vi "Switch_DataLog.vi"() -> ()   [LabVIEW 2016]
uses:
  MGCC_DataLog_global.vi
  Finite State Machine (He Yin)/Sub-VIs/MGCC_FntStaMach_gobal.vi
  Global tdms reference.vi
  Communication/Global communication.vi
  Model Management (He Yin)/Global_MdlMgmt.vi
  <vilib>/Utility/error.llb/Error Cluster From Error Code.vi
  <vilib>/ErrorRing/Error Ring.xnode
panel:
  in  "Start 3":bool=TRUE
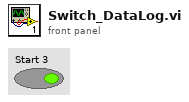
[diagram p1: front panel]
types:
  T1 = enum16{"open", "open or create", "create or replace", "create", "open (read-only)"}
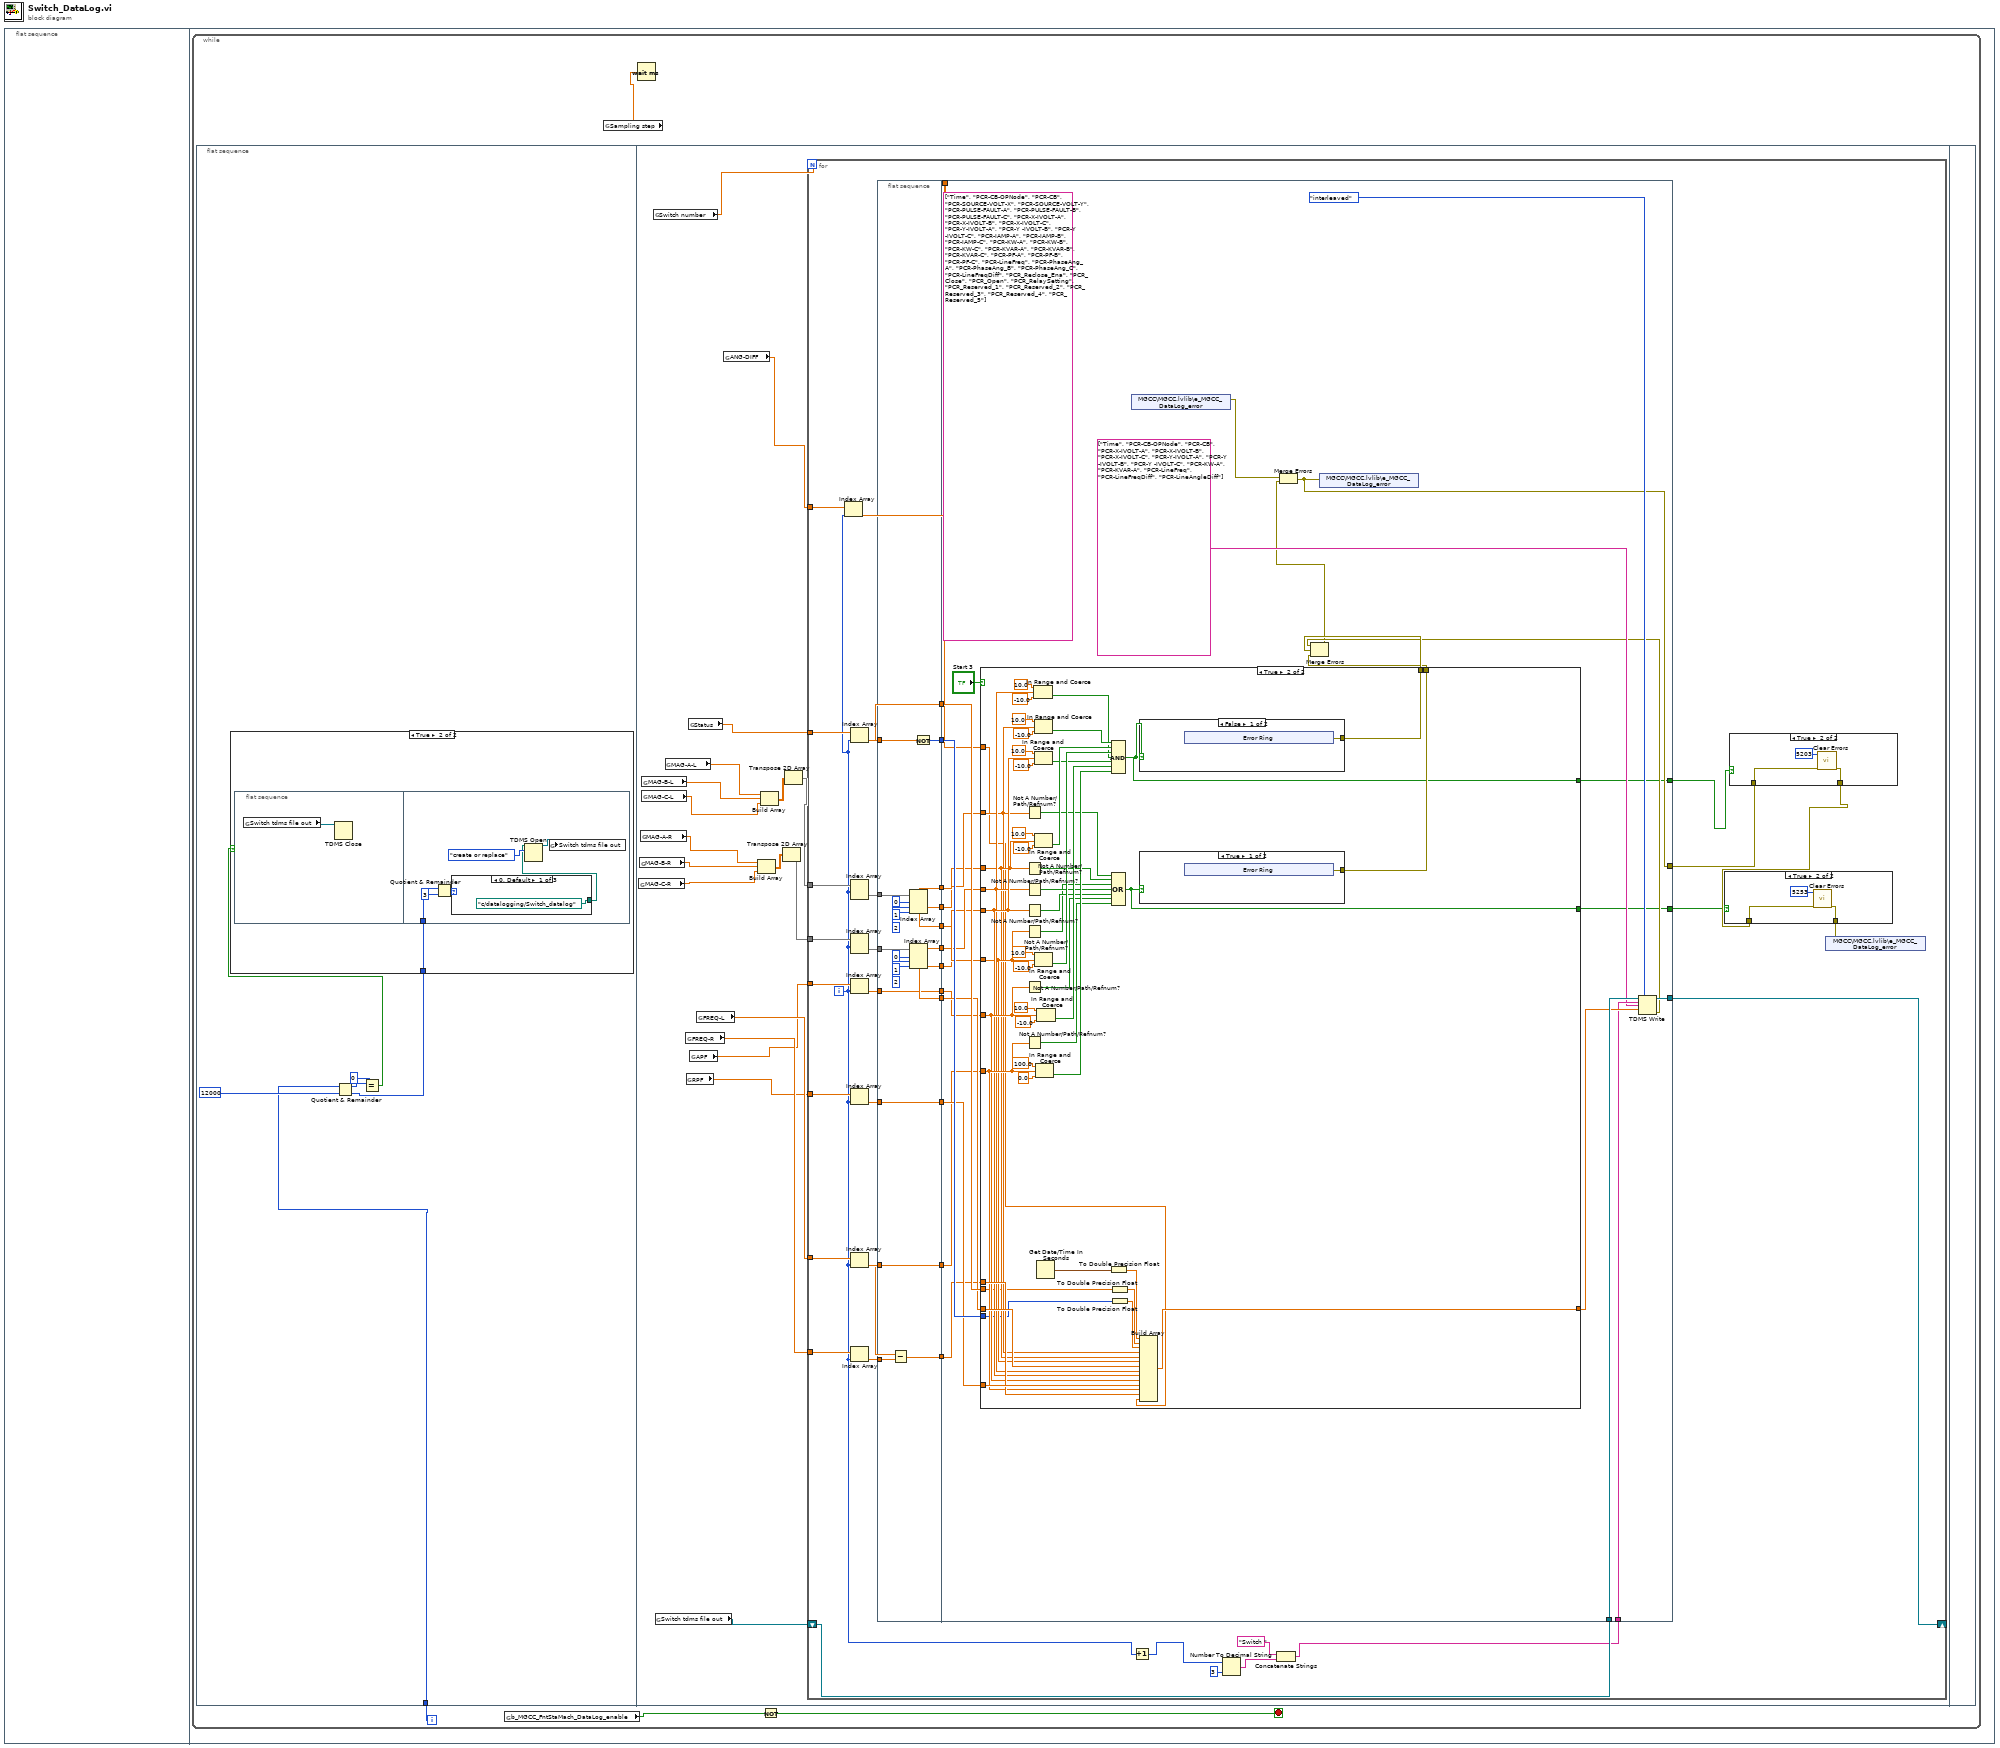
[diagram p0: block diagram]
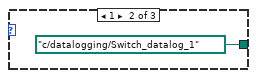
[diagram p3: hidden frame]
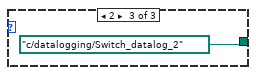
[diagram p4: hidden frame]
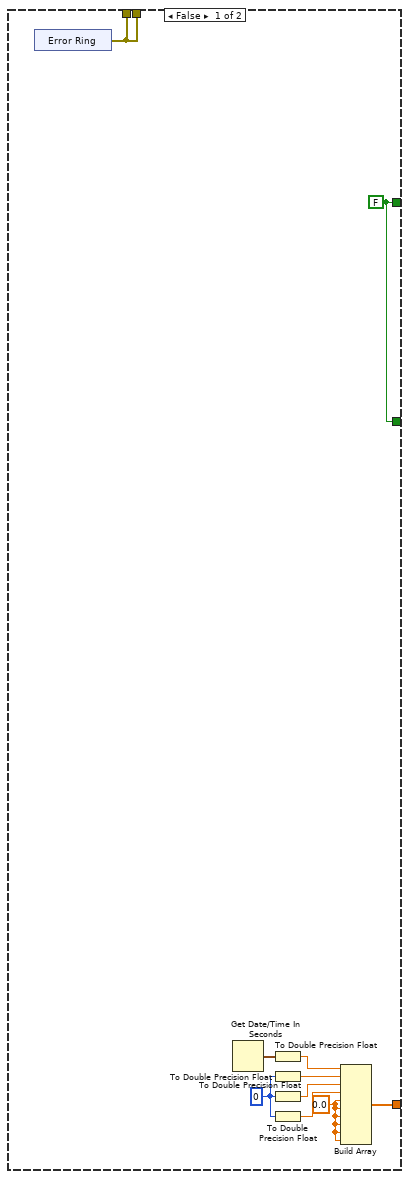
[diagram p7: hidden frame]
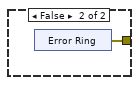
[diagram p8: hidden frame]
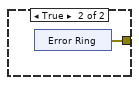
[diagram p9: hidden frame]
diagram:
  n1 = flat-sequence {
    frame #0 {
    }
    frame #1 {
      n2 = while {
        i -> [w2]
        stop <- w4 stop-if-true
        n3 = flat-sequence {
          tunnel: w2 -> [w5]
          frame #0 {
            n4 = Quotient & Remainder(x=w5, y=12000) -> (x-y*floor(x/y)=w9:i32, floor(x/y)=w6:i32)
            n5 = Equal?(x=w9, y=0) -> (x = y?=w7:bool)
            n6 = case shown="True" w7 {
              tunnel: w6 -> [_ w11]
              frame False {
              }
              frame True {
                n7 = flat-sequence {
                  tunnel: w11 -> [w16]
                  frame #0 {
                    n8 = global read "Global tdms reference.vi" "Switch tdms file out"() -> (w12:refnum<k34>)
                    n9 = TDMS Close(11:w12) -> ()  [unwired: 1 in, 2 out]
                  }
                  frame #1 {
                    n10 = Quotient & Remainder(x=w16, y=3) -> (x-y*floor(x/y)=w14:i32)  [unwired: 1 out]
                    n11 = case shown="0, Default" w14 {
                      tunnel: [path "c:/datalogging/Switch_datalog" ("file path (dialog if empty)") path "c:/datalogging/Switch_datalog_1" ("file path (dialog if empty)") path "c:/datalogging/Switch_datalog_2" ("file path (dialog if empty)")] -> w13
                      frame 0, Default {
                      }
                      frame 1 {
                      }
                      frame 2 {
                      }
                    }
                    n12 = TDMS Open(10:T1."create or replace" ("operation (0:open)"), 11:w13) -> (3:w18:refnum<k34>)  [unwired: 5 in, 1 out]
                    n13 = global write "Global tdms reference.vi" "Switch tdms file out"(w18) -> ()
                  }
                }
              }
            }
          }
          frame #1 {
            n14 = global read "Global communication.vi" "MAG-C-R"() -> (w26:dbl[])
            n15 = global read "Global communication.vi" "MAG-B-R"() -> (w27:dbl[])
            n16 = global read "Global communication.vi" "MAG-A-R"() -> (w28:dbl[])
            n17 = global read "Global communication.vi" "MAG-B-L"() -> (w24:dbl[])
            n18 = global read "Global communication.vi" "MAG-C-L"() -> (w23:dbl[])
            n19 = global read "Global_MdlMgmt.vi" "Switch number"() -> (w22:dbl)
            n20 = global read "Global tdms reference.vi" "Switch tdms file out"() -> (w39:refnum<k34>)
            n21 = global read "Global communication.vi" "MAG-A-L"() -> (w25:dbl[])
            n22 = global read "Global communication.vi" "FREQ-R"() -> (w31:dbl[])
            n23 = global read "Global communication.vi" "RPF"() -> (w29:dbl[])
            n24 = global read "Global communication.vi" "Status"() -> (w33:dbl[])
            n25 = global read "Global communication.vi" "APF"() -> (w30:dbl[])
            n26 = global read "Global communication.vi" "FREQ-L"() -> (w32:dbl[])
            n27 = global read "Global communication.vi" "ANG-DIFF"() -> (w34:dbl[])
            n28 = Build Array(w28, w27, w26) -> (w36:dbl[][])
            n29 = Build Array(w25, w24, w23) -> (w38:dbl[][])
            n30 = Transpose 2D Array(2D array=w36) -> (transposed array=w35:dbl[][])
            n31 = Transpose 2D Array(2D array=w38) -> (transposed array=w37:dbl[][])
            n32 = for {
              N: w22 -> [_]
              tunnel: w33 -> [w78]
              tunnel: w37 -> [w74]
              tunnel: w35 -> [w72]
              tunnel: w30 -> [w68]
              tunnel: w29 -> [w70]
              tunnel: w32 -> [w66]
              tunnel: w31 -> [w76]
              shift-right: [w79] -> _
              shift-left: w39 -> [w80]
              tunnel: w34 -> [w50]
              i -> [w44]
              n33 = Index Array(array=w50, index=w44) -> (element=w49:dbl)
              n34 = Index Array(array=w78, index=w44) -> (element=w77:dbl)
              n35 = Index Array(array=w74, index (row)=w44) -> (element=w73:dbl[])  [unwired: 1 in]
              n36 = Index Array(array=w72, index (row)=w44) -> (element=w71:dbl[])  [unwired: 1 in]
              n37 = Index Array(array=w68, index=w44) -> (element=w67:dbl)
              n38 = Index Array(array=w70, index=w44) -> (element=w69:dbl)
              n39 = Index Array(array=w66, index=w44) -> (element=w65:dbl)
              n40 = Index Array(array=w76, index=w44) -> (element=w75:dbl)
              n41 = flat-sequence {
                tunnel: w77 -> [w100]
                tunnel: w73 -> [w109]
                tunnel: w71 -> [w102]
                tunnel: w67 -> [w92]
                tunnel: w69 -> [w91]
                tunnel: w65 -> [w90]
                tunnel: w75 -> [w101]
                tunnel: [w100] -> w64
                tunnel: [w99] -> w63
                tunnel: [w98] -> w62
                tunnel: [w97] -> w61
                tunnel: [w96] -> w60
                tunnel: [w95] -> w59
                tunnel: [w94] -> w58
                tunnel: [w93] -> w57
                tunnel: [w92] -> w56
                tunnel: [w91] -> w55
                tunnel: [w90] -> w54
                tunnel: [w89] -> w53
                tunnel: w80 -> [w136]
                tunnel: w45 -> [w133]
                tunnel: [w132] -> w79
                tunnel: w64 -> [w131]
                tunnel: w63 -> [w130]
                tunnel: w62 -> [w129]
                tunnel: w61 -> [w128]
                tunnel: w60 -> [w127]
                tunnel: w59 -> [w126]
                tunnel: w58 -> [w125]
                tunnel: w57 -> [w124]
                tunnel: w56 -> [w123]
                tunnel: w55 -> [w122]
                tunnel: w54 -> [w121]
                tunnel: w53 -> [w120]
                tunnel: [w113] -> w52
                tunnel: [w112] -> w51
                tunnel: w49 -> [w111]
                tunnel: [w110] -> w40
                frame #0 {
                  n42 = Subtract(x=w90, y=w101) -> (x-y=w89:dbl)
                  n43 = Index Array(array=w109, index #1=0 ("index"), index #2=1 ("index"), index #3=2 ("index")) -> (element #1=w98:dbl, element #2=w97:dbl, element #3=w96:dbl)
                  n44 = Index Array(array=w102, index #1=0 ("index"), index #2=1 ("index"), index #3=2 ("index")) -> (element #1=w95:dbl, element #2=w94:dbl, element #3=w93:dbl)
                  n45 = Not(x=w100) -> (.not. x?=w99:u32)
                }
                frame #1 {
                  (unwired) string[] ["Time", "PCR-CB-OPNode", "PCR-CB", "PCR-SOURCE-VOLT-X", "PCR-SOURCE-VOLT-Y", "PCR-PULSE-FAULT-A", "PCR-PULSE-FAULT-B", "PCR-PULSE-FAULT-C", "PCR-X-IVOLT-A", "PCR-X-IVOLT-B", "PCR-X-IVOLT-C", "PCR-Y-IVOLT-A", "PCR-Y -IVOLT-B", "PCR-Y -IVOLT-C", "PCR-IAMP-A", "PCR-IAMP-B", "PCR-IAMP-C", "PCR-KW-A", "PCR-KW-B", "PCR-KW-C", "PCR-KVAR-A", "PCR-KVAR-B", "PCR-KVAR-C", "PCR-PF-A", "PCR-PF-B", "PCR-PF-C", "PCR-LineFreq", "PCR-PhaseAng_A", "PCR-PhaseAng_B", "PCR-PhaseAng_C", "PCR-LineFreqDiff", "PCR_Reclose_Ena", "PCR_Close", "PCR_Open", "PCR_RelaySetting", "PCR_Reserved_1", "PCR_Reserved_2", "PCR_Reserved_3", "PCR_Reserved_4", "PCR_Reserved_5"] ("channel name(s) in (Untitled)")
                  n46 = case shown="True" "Start 3" {
                    tunnel: [w142 w198] -> w134
                    tunnel: w131 -> [_ w150]
                    tunnel: w130 -> [_ w151]
                    tunnel: w129 -> [_ w156]
                    tunnel: w128 -> [_ w158]
                    tunnel: w127 -> [_ w160]
                    tunnel: w126 -> [_ w193]
                    tunnel: w125 -> [_ w162]
                    tunnel: w124 -> [_ w164]
                    tunnel: w123 -> [_ w166]
                    tunnel: w122 -> [_ w192]
                    tunnel: w121 -> [_ w168]
                    tunnel: w120 -> [_ w191]
                    tunnel: [w139 w169] -> w118
                    tunnel: [w139 w154] -> w115
                    tunnel: [w138 w153] -> w112
                    tunnel: w111 -> [_ w152]
                    tunnel: [w138 w149] -> w110
                    frame False {
                      w138 = FALSE
                      w144 = 0.0
                      w141 = 0
                      n47 = xnode "Error Ring"() -> ("error out"=w139:errorcluster)
                      n48 = Get Date/Time In Seconds() -> (seconds since 1Jan1904=w140:timestamp)
                      n49 = To Double Precision Float(number=w140) -> (double precision float=w143:dbl)
                      n50 = To Double Precision Float(number=w141) -> (double precision float=w147:dbl)
                      n51 = To Double Precision Float(number=w141) -> (double precision float=w146:dbl)
                      n52 = To Double Precision Float(number=w141) -> (double precision float=w145:dbl)
                      n53 = Build Array(w143, w147, w146, w145, w144, w144, w144, w144, w144, w144) -> (w142:dbl[])
                    }
                    frame True {
                      n54 = Not A Number/Path/Refnum?(number/path/refnum=w156) -> (NaN/Path/Refnum?=w155:bool)
                      n55 = Not A Number/Path/Refnum?(number/path/refnum=w158) -> (NaN/Path/Refnum?=w157:bool)
                      n56 = Not A Number/Path/Refnum?(number/path/refnum=w162) -> (NaN/Path/Refnum?=w161:bool)
                      n57 = Not A Number/Path/Refnum?(number/path/refnum=w164) -> (NaN/Path/Refnum?=w163:bool)
                      n58 = Not A Number/Path/Refnum?(number/path/refnum=w160) -> (NaN/Path/Refnum?=w159:bool)
                      n59 = Not A Number/Path/Refnum?(number/path/refnum=w166) -> (NaN/Path/Refnum?=w165:bool)
                      n60 = Not A Number/Path/Refnum?(number/path/refnum=w168) -> (NaN/Path/Refnum?=w167:bool)
                      n61 = In Range and Coerce(upper limit=10.0, x=w162, lower limit=-10.0) -> (In Range?=w173:bool)  [unwired: 1 out]
                      n62 = In Range and Coerce(upper limit=10.0, x=w156, lower limit=-10.0) -> (In Range?=w176:bool)  [unwired: 1 out]
                      n63 = In Range and Coerce(upper limit=10.0, x=w164, lower limit=-10.0) -> (In Range?=w172:bool)  [unwired: 1 out]
                      n64 = In Range and Coerce(upper limit=10.0, x=w158, lower limit=-10.0) -> (In Range?=w175:bool)  [unwired: 1 out]
                      n65 = In Range and Coerce(upper limit=10.0, x=w160, lower limit=-10.0) -> (In Range?=w174:bool)  [unwired: 1 out]
                      n66 = In Range and Coerce(upper limit=100.0, x=w168, lower limit=0.0) -> (In Range?=w170:bool)  [unwired: 1 out]
                      n67 = Get Date/Time In Seconds() -> (seconds since 1Jan1904=w195:timestamp)
                      n68 = In Range and Coerce(upper limit=10.0, x=w166, lower limit=-10.0) -> (In Range?=w171:bool)  [unwired: 1 out]
                      n69 = To Double Precision Float(number=w195) -> (double precision float=w194:dbl)
                      n70 = To Double Precision Float(number=w150) -> (double precision float=w197:dbl)
                      n71 = To Double Precision Float(number=w151) -> (double precision float=w196:dbl)
                      n72 = Compound Arithmetic op=AND(w176, w175, w174, w173, w172, w171, w170) -> (w153:bool)
                      n73 = Compound Arithmetic op=OR(w155, w157, w159, w161, w163, w165, w167) -> (w149:bool)
                      n74 = case shown="False" w153 {
                        tunnel: [w207 w213] -> w169
                        frame False {
                          n75 = xnode "Error Ring"() -> ("error out"=w207:errorcluster)
                        }
                        frame True {
                          n76 = xnode "Error Ring"() -> ("error out"=w213:errorcluster)
                        }
                      }
                      n77 = case shown="True" w149 {
                        tunnel: [w199 w205] -> w154
                        frame True {
                          n78 = xnode "Error Ring"() -> ("error out"=w199:errorcluster)
                        }
                        frame False {
                          n79 = xnode "Error Ring"() -> ("error out"=w205:errorcluster)
                        }
                      }
                      n80 = Build Array(w194, w197, w196, w156, w158, w160, w193, w162, w164, w166, w192, w168, w191, w152) -> (w198:dbl[])
                    }
                  }
                  n81 = shared-variable "MGCC\\MGCC.lvlib\\e_MGCC_DataLog_error"() -> (w116:errorcluster)  [unwired: 1 in, 1 out]
                  n82 = TDMS Write(0:w136, 1:enum16{"decimated", "interleaved"}."interleaved" ("data layout (0:decimated)"), 5:w133, 7:string[] ["Time", "PCR-CB-OPNode", "PCR-CB", "PCR-X-IVOLT-A", "PCR-X-IVOLT-B", "PCR-X-IVOLT-C", "PCR-Y-IVOLT-A", "PCR-Y -IVOLT-B", "PCR-Y -IVOLT-C", "PCR-KW-A", "PCR-KVAR-A", "PCR-LineFreq", "PCR-LineFreqDiff", "PCR-LineAngleDiff"] ("channel name(s) in (Untitled)"), 9:w134) -> (4:w132:refnum<k34>, 15:w117:errorcluster)  [unwired: 1 in, 2 out]
                  n83 = Merge Errors(w117, w118, w115) -> (w114:errorcluster)
                  n84 = Merge Errors(w116, w114) -> (w113:errorcluster)
                  n85 = shared-variable "MGCC\\MGCC.lvlib\\e_MGCC_DataLog_error"(w113) -> ()  [unwired: 1 in, 1 out]
                }
              }
              n86 = Increment(x=w44) -> (x+1=w43:i32)
              n87 = Number To Decimal String(number=w43, width (-)=i16 3) -> (decimal integer string=w46:string)
              n88 = Concatenate Strings("Switch " ("group name in (Untitled)"), w46) -> (w45:string)
              n89 = case shown="True" w51 {
                tunnel: w52 -> [w85 w88]
                tunnel: [w85 w86] -> w41
                frame False {
                }
                frame True {
                  n90 = call <vilib>:"Clear Errors.vi"("error in (no error)"=w88, "specific error code to clear (0: all)"=5203) -> ("error out"=w86:errorcluster)  [unwired: 4 in, 1 out]
                }
              }
              n91 = case shown="True" w40 {
                tunnel: w41 -> [w81 w84]
                tunnel: [w81 w82] -> w42
                frame False {
                }
                frame True {
                  n92 = call <vilib>:"Clear Errors.vi"("error in (no error)"=w84, "specific error code to clear (0: all)"=5253) -> ("error out"=w82:errorcluster)  [unwired: 4 in, 1 out]
                }
              }
              n93 = shared-variable "MGCC\\MGCC.lvlib\\e_MGCC_DataLog_error"(w42) -> ()  [unwired: 1 in, 1 out]
            }
          }
          frame #2 {
          }
        }
        n94 = global read "MGCC_FntStaMach_gobal.vi" "b_MGCC_FntStaMach_DataLog_enable"() -> (w1:bool)
        n95 = global read "MGCC_DataLog_global.vi" "Sampling step"() -> (w3:dbl)
        n96 = Wait (ms)(milliseconds to wait=w3) -> ()  [unwired: 1 out]
        n97 = Not(x=w1) -> (.not. x?=w4:bool)
      }
    }
  }
